vi "prepare airyscam buffer.vi"(7 "buffer page size":i32, 10 "frames":i32, 11 "Camera handle in":u32) -> (0 "buffer pointers":u64[](array[numeric]), 3 "buffer array":T1[](array[typedef]))   [LabVIEW 2015]
uses:
  <vilib>/vision/Image Controls.llb/IMAQ Image.ctl
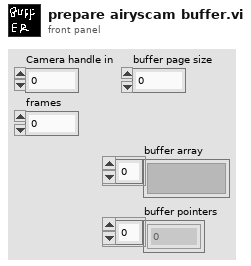
[diagram p1: front panel]
types:
  T1 = typedef "IMAQ Image.ctl" = refnum<image>
  T2 = enum32{"Map Pixel Pointer", "Unmap Pixel Pointer", "Get Pixels Infos"}
  T3 = typedef "Image Type" = u32
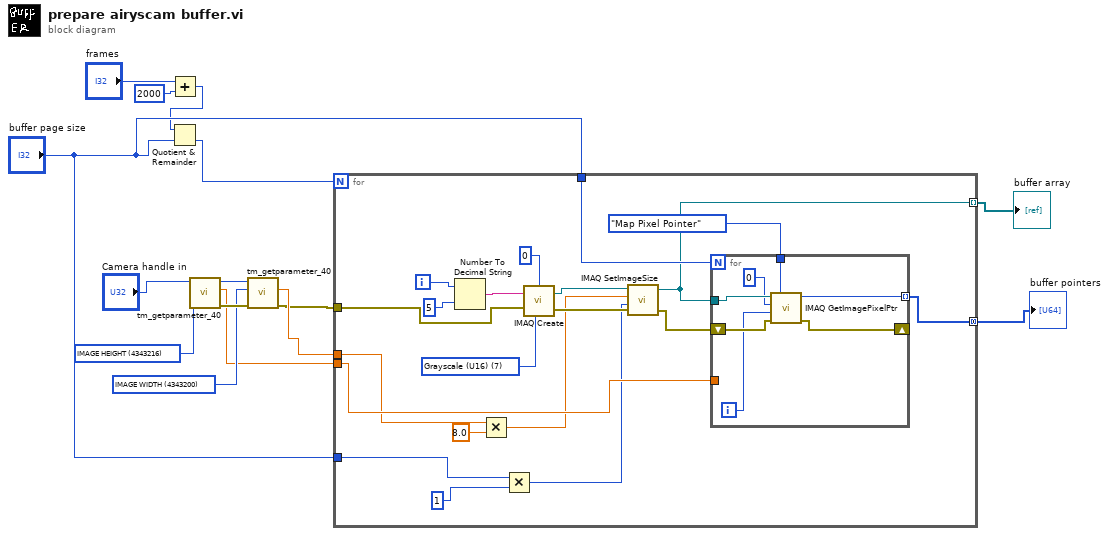
[diagram p0: block diagram]
diagram:
  w11 = u32 4343200 items=["SENSOR MODE"=4212128, "READOUT SPEED"=4211872, "READOUT DIRECTION"=4211904, "TRIGGER GLOBAL EXPOSURE"=2049680, "TRIGGER DELAY"=1066480, "INTERNAL TRIGGER HANDLING"=1066496, "SENSOR TEMPERATURE"=2115232, "SENSOR COOLER STATUS"=2115280, "EXPOSURE TIME"=2049184, "DEFECT CORRECT MODE"=4670368, "HOT PIXEL CORRECT LEVEL"=4670400, "BINNING"=4215968, "TIMING READOUT TIME"=4223904, "INTERNAL FRAME RATE"=4225952, "INTERNAL FRAME INTERVAL"=4225968, "INTERNAL LINE SPEED"=4226000, "INTERNAL LINE INTERVAL"=4226016, "IMAGE WIDTH"=4343200, "IMAGE HEIGHT"=4343216, "IMAGE ROWBYTES"=4343232, "IMAGE FRAMEBYTES"=4343248, "IMAGE PIXEL TYPE"=4343296, "NUMBER OF OUTPUT TRIGGER CONNECTOR"=1852320, "OUTPUT TRIGGER SOURCE[0]"=1852576, "OUTPUT TRIGGER SOURCE[1]"=1852832, "OUTPUT TRIGGER SOURCE[2]"=1853088, "OUTPUT TRIGGER POLARITY[0]"=1852592, "OUTPUT TRIGGER POLARITY[1]"=1852848, "OUTPUT TRIGGER POLARITY[2]"=1853104, "OUTPUT TRIGGER ACTIVE[0]"=1852608, "OUTPUT TRIGGER ACTIVE[1]"=1852864, "OUTPUT TRIGGER ACTIVE[2]"=1853120, "OUTPUT TRIGGER DELAY[0]"=1852624, "OUTPUT TRIGGER DELAY[1]"=1852880, "OUTPUT TRIGGER DELAY[2]"=1853136, "OUTPUT TRIGGER PERIOD[0]"=1852640, "OUTPUT TRIGGER PERIOD[1]"=1852896, "OUTPUT TRIGGER PERIOD[2]"=1853152, "OUTPUT TRIGGER KIND[0]"=1852656, "OUTPUT TRIGGER KIND[1]"=1852912, "OUTPUT TRIGGER KIND[2]"=1853168, "OUTPUT TRIGGER BASE SENSOR[0]"=1852672, "OUTPUT TRIGGER BASE SENSOR[1]"=1852928, "OUTPUT TRIGGER BASE SENSOR[2]"=1853184, "OUTPUT TRIGGER PRE HSYNC COUNT"=1852704] ("Parameter")
  w12 = u32 4343216 items=["SENSOR MODE"=4212128, "READOUT SPEED"=4211872, "READOUT DIRECTION"=4211904, "TRIGGER GLOBAL EXPOSURE"=2049680, "TRIGGER DELAY"=1066480, "INTERNAL TRIGGER HANDLING"=1066496, "SENSOR TEMPERATURE"=2115232, "SENSOR COOLER STATUS"=2115280, "EXPOSURE TIME"=2049184, "DEFECT CORRECT MODE"=4670368, "HOT PIXEL CORRECT LEVEL"=4670400, "BINNING"=4215968, "TIMING READOUT TIME"=4223904, "INTERNAL FRAME RATE"=4225952, "INTERNAL FRAME INTERVAL"=4225968, "INTERNAL LINE SPEED"=4226000, "INTERNAL LINE INTERVAL"=4226016, "IMAGE WIDTH"=4343200, "IMAGE HEIGHT"=4343216, "IMAGE ROWBYTES"=4343232, "IMAGE FRAMEBYTES"=4343248, "IMAGE PIXEL TYPE"=4343296, "NUMBER OF OUTPUT TRIGGER CONNECTOR"=1852320, "OUTPUT TRIGGER SOURCE[0]"=1852576, "OUTPUT TRIGGER SOURCE[1]"=1852832, "OUTPUT TRIGGER SOURCE[2]"=1853088, "OUTPUT TRIGGER POLARITY[0]"=1852592, "OUTPUT TRIGGER POLARITY[1]"=1852848, "OUTPUT TRIGGER POLARITY[2]"=1853104, "OUTPUT TRIGGER ACTIVE[0]"=1852608, "OUTPUT TRIGGER ACTIVE[1]"=1852864, "OUTPUT TRIGGER ACTIVE[2]"=1853120, "OUTPUT TRIGGER DELAY[0]"=1852624, "OUTPUT TRIGGER DELAY[1]"=1852880, "OUTPUT TRIGGER DELAY[2]"=1853136, "OUTPUT TRIGGER PERIOD[0]"=1852640, "OUTPUT TRIGGER PERIOD[1]"=1852896, "OUTPUT TRIGGER PERIOD[2]"=1853152, "OUTPUT TRIGGER KIND[0]"=1852656, "OUTPUT TRIGGER KIND[1]"=1852912, "OUTPUT TRIGGER KIND[2]"=1853168, "OUTPUT TRIGGER BASE SENSOR[0]"=1852672, "OUTPUT TRIGGER BASE SENSOR[1]"=1852928, "OUTPUT TRIGGER BASE SENSOR[2]"=1853184, "OUTPUT TRIGGER PRE HSYNC COUNT"=1852704] ("Parameter")
  n1 = Add(x="frames", y=2000) -> (x+y=w2:i32)
  n2 = Quotient & Remainder(x=w2, y="buffer page size") -> (floor(x/y)=w7:i32)  [unwired: 1 out]
  n3 = call <userlib>:"tm_getparameter_40.vi"("Parameter"=w12, "Handle in"="Camera handle in") -> ("error out"=w14:errorcluster, "Value out"=w10:dbl, "Handle out"=w13:u32)  [unwired: 7 in]
  n4 = call <userlib>:"tm_getparameter_40.vi"("error in (no error)"=w14, "Parameter"=w11, "Handle in"=w13) -> ("error out"=w8:errorcluster, "Value out"=w9:dbl)  [unwired: 6 in, 1 out]
  n5 = for {
    N: w7 -> [_]
    tunnel: w10 -> [w21]
    tunnel: w9 -> [w19]
    tunnel: w8 -> [w24]
    tunnel: "buffer page size" -> [w29]
    tunnel: [w27] -> w6 mode=concatenating
    tunnel: [w26] -> w5 mode=indexing
    tunnel: "buffer page size" -> [w22]
    i -> [w35]
    w32 = T3 7 items=["Grayscale (U8)", "Grayscale (I16)", "Grayscale (SGL)", "Complex (CSG)", "RGB (U32)", "HSL (U32)", "RGB (U64)", "Grayscale (U16)"] ("Image Type")
    n6 = Number To Decimal String(number=w35, width (-)=5) -> (decimal integer string=w33:string)
    n7 = Multiply(x=w19, y=8.0) -> (x*y=w17:dbl)
    n8 = Multiply(x=w22, y=1) -> (x*y=w20:i32)
    n9 = call "IMAQ Create"("Border Size"=0, "Image Name"=w33, "Image Type"=w32, "error in (no error)"=w24) -> ("New Image"=w30:T1, "error out"=w23:errorcluster)  [unwired: 1 in]
    n10 = call "IMAQ SetImageSize"("error in (no error)"=w23, "Y Resolution"=w20, "X Resolution"=w17, "Image"=w30) -> ("error out"=w28:errorcluster, "Image Out"=w26:T1)  [unwired: 1 in]
    n11 = for {
      N: w29 -> [_]
      tunnel: w26 -> [w42]
      shift-right: [w40] -> _
      shift-left: w28 -> [w41]
      tunnel: w21 -> [_]
      tunnel: [w38] -> w27 mode=indexing
      tunnel: T2."Map Pixel Pointer" ("Function") -> [w37]
      i -> [w36]
      n12 = call "IMAQ GetImagePixelPtr"("Function"=w37, "error in (no error)"=w41, "Y Coordinate"=w36, "X Coordinate"=0, "Image"=w42) -> ("error out"=w40:errorcluster, "Pixel Pointer out"=w38:u64)  [unwired: 1 in, 4 out]
    }
  }
  "buffer array" <- w5
  "buffer pointers" <- w6
